vi "Barcode Example.vi"() -> ()   [LabVIEW 2011]
doc: "This example shows how to use the IMAQ Read Barcode VI to read standard 1D barcodes."
uses:
  <vilib>/vision/NI_Vision_Development_Module.lvlib
panel:
  out "Image":T1(plugin-control) caption="Draw a Rectangular Region of Interest on the BarCode"
  out "Code":string
  in  "Delay (ms)":i32(slide)=1446 max=3000 scale=0.0..2000.0
  in  "stop":bool
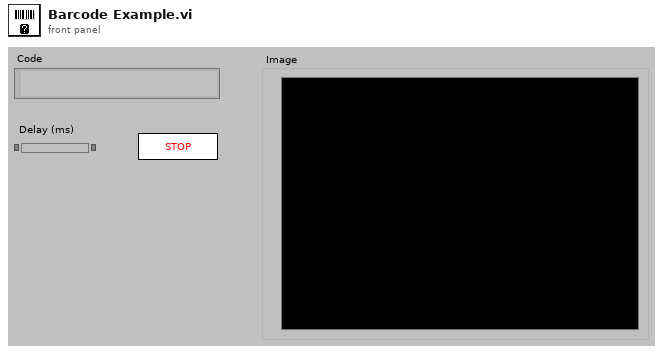
[diagram p1: front panel]
types:
  T1 = typedef "IMAQ Image.ctl" = refnum<image>
  T2 = cluster{i32[], cluster{"Contour Type":u32, "ROI Type":u32, i32[]}[]}
  T3 = cluster{"Special Char 1":string, "Special Char 2":string, "Confidence Level":sgl, "Barcode Type":u32}
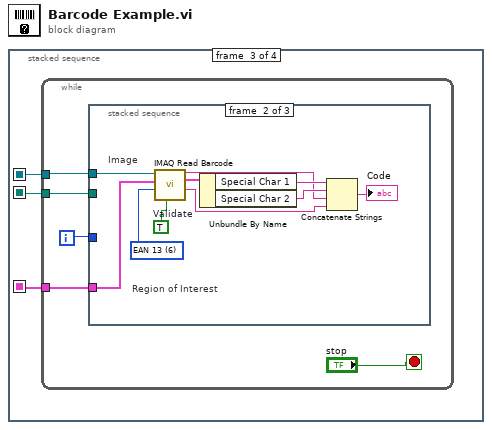
[diagram p0: block diagram]
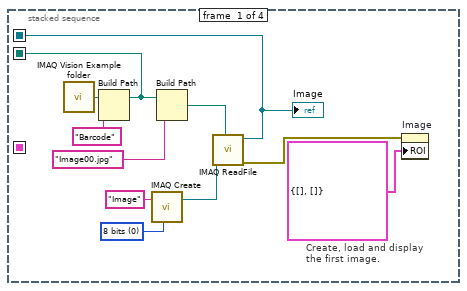
[diagram p2: hidden frame]
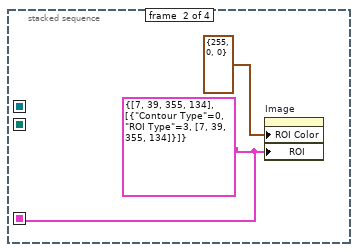
[diagram p3: hidden frame]
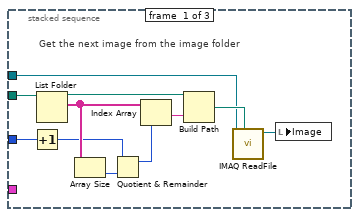
[diagram p4: hidden frame]
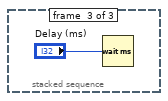
[diagram p5: hidden frame]
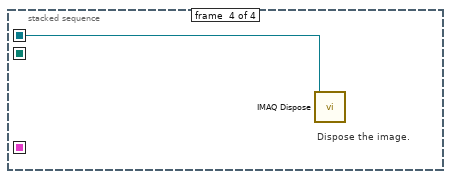
[diagram p6: hidden frame]
diagram:
  n1 = stacked-sequence {
    seq-local: [w4 _ _ _] -> [_ _ w15 w44]
    seq-local: [_ w12 _ _] -> [_ _ w16 _]
    seq-local: [w6 _ _ _] -> [_ _ w14 _]
    frame #0 {
      w5 = u32 0 items=["8 bits", "16 bits", "Float", "Complex", "RGB", "HSL"] ("Image Type")
      # "Create, load and display the first image."
      n2 = call "IMAQ Vision Example folder.vi"() -> ("Example Image Path"=w1:path)  [unwired: 1 out]
      n3 = Build Path(base path=w1, name or relative path="Barcode") -> (appended path=w6:path)
      n4 = call "IMAQ Create"("Image Name"="Image", "Image Type"=w5) -> ("New Image"=w8:T1)  [unwired: 2 in, 2 out]
      n5 = Build Path(base path=w6, name or relative path="Image00.jpg") -> (appended path=w7:path)
      n6 = call "IMAQ ReadFile"("File Path"=w7, "Image"=w8) -> ("error out"=w2:errorcluster, "Image Out"=w4:T1)  [unwired: 3 in, 5 out]
      "Image" <- w4
      n7 = property on="Image" class="ImageControl"(error in=w2, "ROI"=T2 {[], []}) -> ()  [unwired: 1 in, 2 out]
    }
    frame #1 {
      w12 = T2 {[7, 39, 355, 134], [{"Contour Type"=0, "ROI Type"=3, [7, 39, 355, 134]}]} ("ROI")
      n8 = property on="Image" class="ImageControl"("ROI Color"=cluster{"Red":u8, "Green":u8, "Blue":u8} {"Red"=255, "Green"=0, "Blue"=0}, "ROI"=w12) -> ()  [unwired: 2 in, 2 out]
    }
    frame #2 {
      n9 = while {
        tunnel: w14 -> [w19]
        tunnel: w15 -> [w20]
        tunnel: w16 -> [w21]
        i -> [w18]
        stop <- "stop" stop-if-true
        n10 = stacked-sequence {
          tunnel: w21 -> [_ w42 _]
          tunnel: w20 -> [w23 w41 _]
          tunnel: w19 -> [w26 _ _]
          tunnel: w18 -> [w24 _ _]
          frame #0 {
            # "Get the next image from the image folder"
            n11 = Increment(x=w24) -> (x+1=w25:i32)
            n12 = List Folder(path=w26) -> (path out=w28:path, filenames=w32:string[])  [unwired: 1 in, 4 out]
            n13 = Array Size(array=w32) -> (size(s)=w31:i32)
            n14 = Quotient & Remainder(x=w25, y=w31) -> (x-y*floor(x/y)=w30:i32)  [unwired: 1 out]
            n15 = Index Array(array=w32, index=w30) -> (element=w29:string)
            n16 = Build Path(base path=w28, name or relative path=w29) -> (appended path=w27:path)
            n17 = call "IMAQ ReadFile"("File Path"=w27, "Image"=w23) -> ("Image Out"=w22:T1)  [unwired: 3 in, 6 out]
            n18 = local write "Image"(w22) -> ()
          }
          frame #1 {
            w34 = TRUE  # Validate
            w40 = u32 6 items=["Reserved", "Codabar", "Code 39", "Code 93", "Code 128", "EAN 8", "EAN 13", "Interleaved 2 of 5", "MSI", "UPCA"] ("Barcode Type")
            # "Region of Interest"
            # "Image"
            n19 = call "IMAQ Read Barcode"("Validate"=w34, "Barcode Type"=w40, "ROI Descriptor"=w42, "Image"=w41) -> ("Checksum(s)"=w33:string, "Extra Info"=w39:T3, "String"=w36:string)  [unwired: 1 in, 4 out]
            n20 = Unbundle By Name(w39) -> ("Special Char 1"=w38:string, "Special Char 2"=w37:string)
            n21 = Concatenate Strings(w38, w37, w36, w33) -> (→"Code":string)
          }
          frame #2 {
            n22 = Wait (ms)(milliseconds to wait="Delay (ms)") -> ()  [unwired: 1 out]
          }
        }
      }
    }
    frame #3 {
      # "Dispose the image."
      n23 = call "IMAQ Dispose"("Image"=w44) -> ()  [unwired: 2 in, 4 out]
    }
  }
